vi "Save Stimulus File Name (SubVI).vi"(11 "Stimulus File Name":path) -> ()   [LabVIEW 2020]
uses:
  <vilib>/Utility/config.llb/Write Key (String).vi
  <vilib>/Utility/config.llb/NI_LVConfig.lvlib
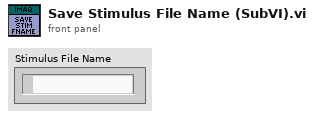
[diagram p1: front panel]
types:
  T1 = typedef "NI_LVConfig.lvlib/Config Data RefNum.ctl" = refnum<k1>
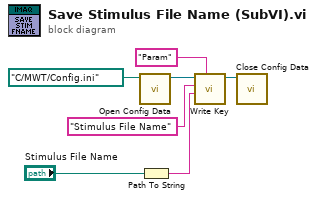
[diagram p0: block diagram]
diagram:
  n1 = call <vilib>:"Open Config Data.vi"("configuration file path"=path "C:/MWT/Config.ini") -> ("refnum"=w7:T1)  [unwired: 8 in, 2 out]
  n2 = Path To String(path="Stimulus File Name") -> (string=w1:string)
  n3 = call-poly <vilib>:"Write Key.vi"("section"="Param", "value"=w1, "key"="Stimulus File Name" ("section"), "refnum"=w7) -> ("refnum out"=w5:T1)  [unwired: 5 in, 2 out]
  n4 = call <vilib>:"Close Config Data.vi"("refnum"=w5) -> ()  [unwired: 9 in, 2 out]
